vi "Write Case ID.vi"(8 "error in (no error)":errorcluster, 10 "Case ID":string, 11 "Consumer Msg in":refnum<class "Consumer Msg.lvclass">) -> (0 "error out":errorcluster, 3 "Consumer Msg out":refnum<class "Consumer Msg.lvclass">)   [LabVIEW 2026, in "TALOS.lvlib" / "Father of all uServices.lvlib" / "Consumer Msg.lvclass"]
uses:
  Consumer Msg.lvclass
  Consumer Msg.lvclass/Consumer Msg.ctl
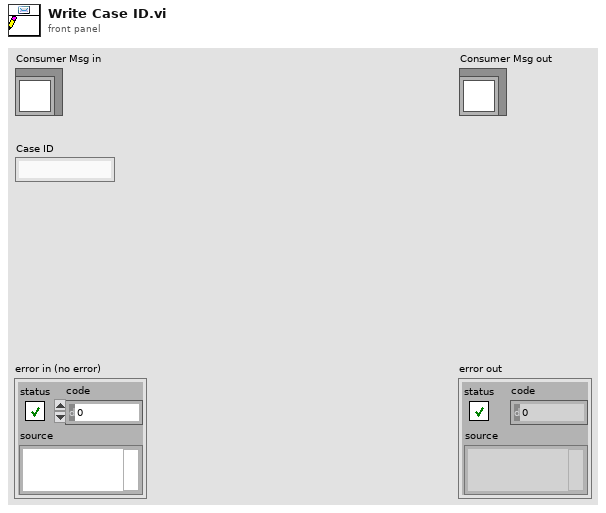
[diagram p1: front panel]
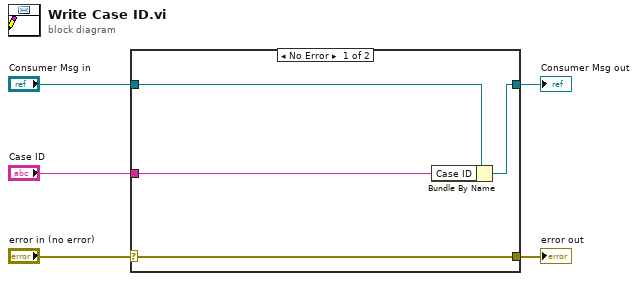
[diagram p0: block diagram]
diagram:
  n1 = case shown="No Error" "error in (no error)" {
    selector: "error in (no error)" -> [w9 w10]
    tunnel: [w9 w10] -> w4
    tunnel: [w7 w11] -> w2
    tunnel: "Consumer Msg in" -> [w8 w11]
    tunnel: "Case ID" -> [w6 _]
    frame No Error {
      n2 = Bundle By Name(cluster=w8, "Case ID"=w6) -> (w7:refnum<class "Consumer Msg.lvclass">)
    }
    frame Error {
    }
  }
  "error out" <- w4
  "Consumer Msg out" <- w2
